vi "Vision Processing.vi"(4 "error in (no error)":errorcluster) -> ()   [LabVIEW 2019]
doc: "This VI runs in parallel to other tasks. It gets images from the camera, processes them for color or shape and use that information to affect robot behavior."
uses:
  <vilib>/Rock Robotics/WPI/Camera/WPI_CameraWhite Balance Values.ctl
  <vilib>/Rock Robotics/WPI/Camera/WPI_CameraFrameRate.ctl
  <vilib>/Rock Robotics/WPI/Camera/WPI_CameraImageSize.ctl
  Robot Global Data.vi
  <vilib>/Rock Robotics/Network Tables/NT Write Number.vi
  <vilib>/Rock Robotics/Network Tables/NT Read Number.vi
  <vilib>/Rock Robotics/Network Tables/NT Write Boolean.vi
panel:
  out "LimeLight":T1
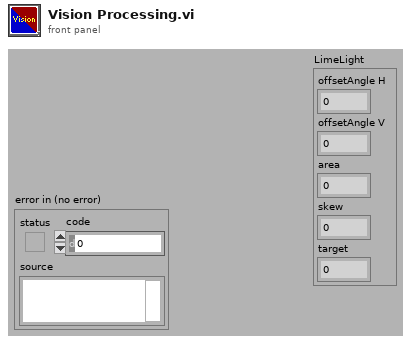
[diagram p1: front panel]
types:
  T1 = cluster{"offsetAngle H":dbl, "offsetAngle V":dbl, "area":dbl, "skew":dbl, "target":dbl}
  T2 = typedef "WPI_CameraImageSize.ctl" = enum16{"640x480", "320x240", "160x120", "Custom"}
  T3 = typedef "WPI_CameraFrameRate.ctl" = u32
  T4 = typedef "WPI_CameraWhite Balance Values.ctl" = enum16{"Auto", "Fixed indoor", "Fixed outdoor 1", "Fixed outdoor 2", "Fixed fluorescent 1", "Fixed fluorescent 2", "Hold current", "Custom"}
  T5 = typedef "WPI_DigitalInputDevRef.ctl" = cluster{"DevStatus":errorcluster, "DIO Channel":T6}
  T6 = typedef "FPGA_DIOChannel.ctl" = enum8{"DIO 0", "DIO 1", "DIO 2", "DIO 3", "DIO 4", "DIO 5", "DIO 6", "DIO 7", "DIO 8", "DIO 9", "DIO MXP 0", "DIO MXP 1", "DIO MXP 2", "DIO MXP 3", "DIO MXP 4", "DIO MXP 5", "DIO MXP 6", "DIO MXP 7", "DIO MXP 8", "DIO MXP 9", "DIO MXP 10", "DIO MXP 11", "DIO MXP 12", "DIO MXP 13", "DIO MXP 14", "DIO MXP 15", "SPI Port CS1", "SPI Port CS2", "SPI Port CS3", "SPI Port MISO", "SPI Port MOSI", "Invalid"}
  T7 = typedef "WPI_AnalogChannelDevRef.ctl" = cluster{"DevStatus":errorcluster, "Analog Channel":T8}
  T8 = typedef "FPGA_AIChannel.ctl" = enum8{"AI 0", "AI 1", "AI 2", "AI 3", "AI MXP 0", "AI MXP 1", "AI MXP 2", "AI MXP 3", "Invalid"}
  T9 = typedef "WPI_CameraDevRef.ctl" = cluster{"Camera Address":string, "CameraStatus":errorcluster}
  T10 = typedef "Image Type" = u32
  T11 = typedef "IMAQ Image.ctl" = refnum<image>
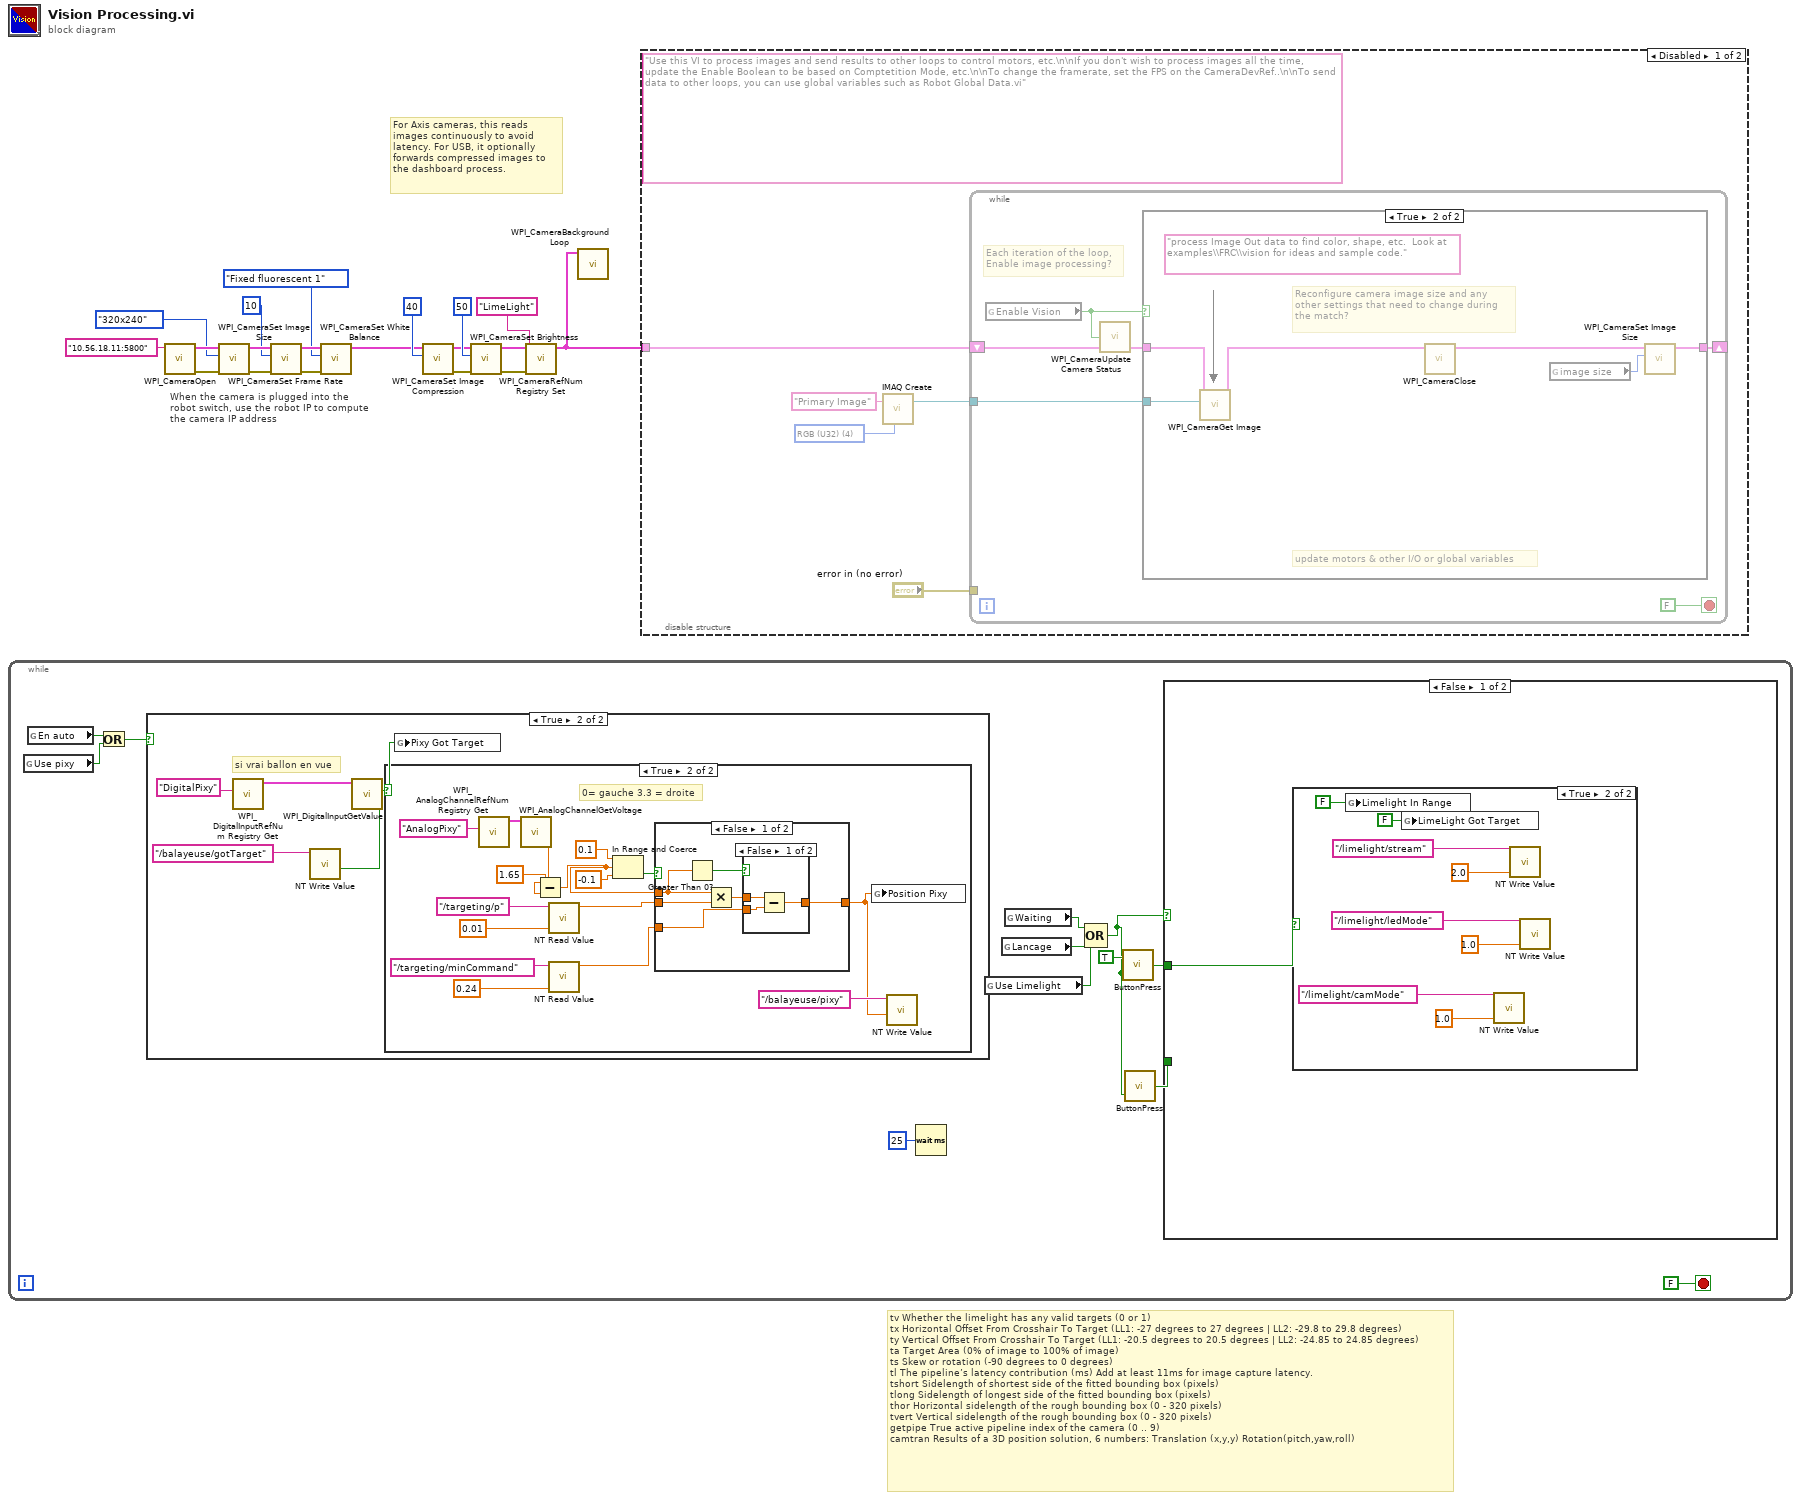
[diagram p0: block diagram]
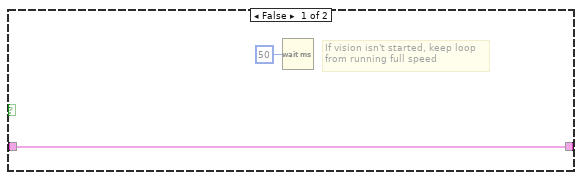
[diagram p2: hidden frame]
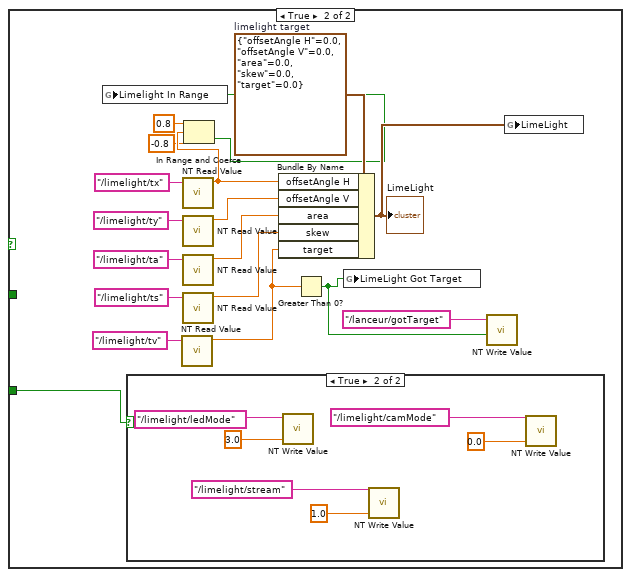
[diagram p5: hidden frame]
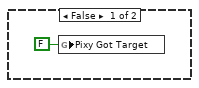
[diagram p7: hidden frame]
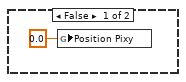
[diagram p8: hidden frame]
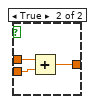
[diagram p9: hidden frame]
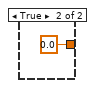
[diagram p10: hidden frame]
diagram:
  # "When the camera is plugged into the\nrobot switch, use the robot IP to compute\nthe camera IP address"
  # "For Axis cameras, this reads\nimages continuously to avoid\nlatency. For USB, it optionally\nforwards compressed images to\nthe dashboard process."
  # "tv\tWhether the limelight has any valid targets (0 or 1)\ntx\tHorizontal Offset From Crosshair To Target (LL1: -27 degrees to 27 degrees | LL2: -29.8 to 29.8 degrees)\nty\tVertical Offset From Crosshair To Target (LL1: -20.5 degrees to 20.5 degrees | LL2: -24.85 to 24.85 degrees)\nta\tTarget Area (0% of image to 100% of image)\nts\tSkew or rotation (-90 degrees to 0 degrees)\ntl\tThe pipeline’s latency contribution (ms) Add at least 11ms for image capture latency.\ntshort\tSidelength of shortest side of the fitted bounding box (pixels)\ntlong\tSidelength of longest side of the fitted bounding box (pixels)\nthor\tHorizontal sidelength of the rough bounding box (0 - 320 pixels)\ntvert\tVertical sidelength of the rough bounding box (0 - 320 pixels)\ngetpipe\tTrue active pipeline index of the camera (0 .. 9)\ncamtran\tResults of a 3D position solution, 6 numbers: Translation (x,y,y) Rotation(pitch,yaw,roll)"
  n1 = while {
    stop <- FALSE stop-if-true
    n2 = global read "Robot Global Data.vi" "Use pixy"() -> (w26:bool)
    n3 = global read "Robot Global Data.vi" "En auto"() -> (w25:bool)
    n4 = Or(x=w25, y=w26) -> (x .or. y?=w24:bool)
    n5 = case shown="True" w24 {
      frame False {
        n6 = global write "Robot Global Data.vi" "Pixy Got Target"(FALSE ("Pixy Got Target")) -> ()
      }
      frame True {
        # "si vrai ballon en vue"
        n7 = call <vilib>:"WPI_DigitalInputRefNum Registry Get.vi"("refnum name"="DigitalPixy") -> ("DigitalInputDevRef"=w69:T5)  [unwired: 9 in, 1 out]
        n8 = call <vilib>:"WPI_DigitalInputGetValue.vi"("DigitalInputDevRef"=w69) -> ("Value"=w67:bool)  [unwired: 8 in, 2 out]
        n9 = call-poly <vilib>:"NT Write Value.vi"("Boolean"=w67, "Name"="/balayeuse/gotTarget") -> ()  [unwired: 9 in, 1 out]
        n10 = case shown="True" w67 {
          frame False {
            n11 = global write "Robot Global Data.vi" "Position Pixy"(0.0 ("Position Pixy")) -> ()
          }
          frame True {
            # "0= gauche 3.3 = droite"
            n12 = call <vilib>:"WPI_AnalogChannelRefNum Registry Get.vi"("refnum name"="AnalogPixy") -> ("AIDeviceRef"=w86:T7)  [unwired: 9 in, 1 out]
            n13 = call <vilib>:"WPI_AnalogChannelGetVoltage.vi"("AIDeviceRef"=w86) -> ("Voltage"=w81:dbl)  [unwired: 8 in, 2 out]
            n14 = Subtract(x=w81, y=1.65) -> (x-y=w79:dbl)
            n15 = call-poly <vilib>:"NT Read Value.vi"("Default Value"=0.01, "Name"="/targeting/p") -> ("Numeric"=w72:dbl)  [unwired: 8 in, 1 out]
            n16 = call-poly <vilib>:"NT Read Value.vi"("Default Value"=0.24, "Name"="/targeting/minCommand") -> ("Numeric"=w71:dbl)  [unwired: 8 in, 1 out]
            n17 = In Range and Coerce(upper limit=0.1, x=w79, lower limit=-0.1) -> (In Range?=w82:bool)  [unwired: 1 out]
            n18 = case shown="False" w82 {
              tunnel: [w90 0.0] -> w77
              tunnel: w79 -> [w89 _]
              tunnel: w72 -> [w88 _]
              tunnel: w71 -> [w87 _]
              frame False {
                n19 = Greater Than 0?(x=w89) -> (x > 0?=w92:bool)
                n20 = Multiply(x=w89, y=w88) -> (x*y=w91:dbl)
                n21 = case shown="False" w92 {
                  tunnel: w91 -> [w95 w98]
                  tunnel: w87 -> [w94 w97]
                  tunnel: [w93 w96] -> w90
                  frame False {
                    n22 = Subtract(x=w95, y=w94) -> (x-y=w93:dbl)
                  }
                  frame True {
                    n23 = Add(x=w98, y=w97) -> (x+y=w96:dbl)
                  }
                }
              }
              frame True {
              }
            }
            n24 = global write "Robot Global Data.vi" "Position Pixy"(w77) -> ()
            n25 = call-poly <vilib>:"NT Write Value.vi"("Numeric"=w77, "Name"="/balayeuse/pixy") -> ()  [unwired: 9 in, 1 out]
          }
        }
        n26 = global write "Robot Global Data.vi" "Pixy Got Target"(w67) -> ()
      }
    }
    n27 = Wait (ms)(milliseconds to wait=u32 25) -> ()  [unwired: 1 out]
    n28 = global read "Robot Global Data.vi" "Use Limelight"() -> (w20:bool)
    n29 = global read "Robot Global Data.vi" "Lancage"() -> (w23:bool)
    n30 = global read "Robot Global Data.vi" "Waiting"() -> (w22:bool)
    n31 = Compound Arithmetic op=OR(w22, w23, w20) -> (w21:bool)
    n32 = call "ButtonPress.vi"("Input"=w21, "Falling Edge?"=TRUE) -> ("Output"=w28:bool)
    n33 = call "ButtonPress.vi"("Input"=w21) -> ("Output"=w27:bool)  [unwired: 1 in]
    n34 = case shown="False" w21 {
      tunnel: w28 -> [w32 _]
      tunnel: w27 -> [_ w47]
      frame False {
        n35 = case shown="True" w32 {
          frame False {
          }
          frame True {
            n36 = global write "Robot Global Data.vi" "Limelight In Range"(FALSE ("LimeLight Got Target")) -> ()
            n37 = global write "Robot Global Data.vi" "LimeLight Got Target"(FALSE ("LimeLight Got Target")) -> ()
            n38 = call-poly <vilib>:"NT Write Value.vi"("Numeric"=1.0, "Name"="/limelight/camMode") -> ()  [unwired: 9 in, 1 out]
            n39 = call-poly <vilib>:"NT Write Value.vi"("Numeric"=2.0, "Name"="/limelight/stream") -> ()  [unwired: 9 in, 1 out]
            n40 = call-poly <vilib>:"NT Write Value.vi"("Numeric"=1.0, "Name"="/limelight/ledMode") -> ()  [unwired: 9 in, 1 out]
          }
        }
      }
      frame True {
        w54 = T1 {"offsetAngle H"=0.0, "offsetAngle V"=0.0, "area"=0.0, "skew"=0.0, "target"=0.0}  # limelight target
        n41 = case shown="True" w47 {
          frame False {
          }
          frame True {
            n42 = call-poly <vilib>:"NT Write Value.vi"("Numeric"=3.0, "Name"="/limelight/ledMode") -> ()  [unwired: 9 in, 1 out]
            n43 = call-poly <vilib>:"NT Write Value.vi"("Numeric"=1.0, "Name"="/limelight/stream") -> ()  [unwired: 9 in, 1 out]
            n44 = call-poly <vilib>:"NT Write Value.vi"("Numeric"=0.0, "Name"="/limelight/camMode") -> ()  [unwired: 9 in, 1 out]
          }
        }
        n45 = call-poly <vilib>:"NT Read Value.vi"("Name"="/limelight/tv") -> ("Numeric"=w48:dbl)  [unwired: 9 in, 1 out]
        n46 = call-poly <vilib>:"NT Read Value.vi"("Name"="/limelight/tx") -> ("Numeric"=w44:dbl)  [unwired: 9 in, 1 out]
        n47 = call-poly <vilib>:"NT Read Value.vi"("Name"="/limelight/ty") -> ("Numeric"=w53:dbl)  [unwired: 9 in, 1 out]
        n48 = call-poly <vilib>:"NT Read Value.vi"("Name"="/limelight/ta") -> ("Numeric"=w52:dbl)  [unwired: 9 in, 1 out]
        n49 = call-poly <vilib>:"NT Read Value.vi"("Name"="/limelight/ts") -> ("Numeric"=w51:dbl)  [unwired: 9 in, 1 out]
        n50 = In Range and Coerce(upper limit=0.8, x=w44, lower limit=-0.8) -> (In Range?=w41:bool)  [unwired: 1 out]
        n51 = global write "Robot Global Data.vi" "Limelight In Range"(w41) -> ()
        n52 = Bundle By Name(cluster=w54, "offsetAngle H"=w44, "offsetAngle V"=w53, "area"=w52, "skew"=w51, "target"=w48) -> (w49:T1)
        "LimeLight" <- w49
        n53 = Greater Than 0?(x=w48) -> (x > 0?=w45:bool)
        n54 = global write "Robot Global Data.vi" "LimeLight Got Target"(w45) -> ()
        n55 = call-poly <vilib>:"NT Write Value.vi"("Boolean"=w45, "Name"="/lanceur/gotTarget") -> ()  [unwired: 9 in, 1 out]
        n56 = global write "Robot Global Data.vi" "LimeLight"(w49) -> ()
      }
    }
  }
  n57 = call <vilib>:"WPI_CameraOpen.vi"("Camera Address"="10.56.18.11:5800" ("format string")) -> ("error out"=w11:errorcluster, "CameraDevRef"=w12:T9)  [unwired: 1 in, 8 out]
  n58 = call <vilib>:"WPI_CameraSet Image Size.vi"("error in (no error)"=w11, "Image Size"=WPI_CameraImageSize."320x240", "CameraDevRef"=w12) -> ("error out"=w10:errorcluster, "CameraDevRef Out"=w13:T9)  [unwired: 1 in, 6 out]
  n59 = call <vilib>:"WPI_CameraSet Frame Rate.vi"("error in (no error)"=w10, "Frame Rate (fps)"=T3 10, "CameraDevRef"=w13) -> ("error out"=w9:errorcluster, "CameraDevRef Out"=w14:T9)  [unwired: 7 out]
  n60 = call <vilib>:"WPI_CameraSet White Balance.vi"("error in (no error)"=w9, "White Balance"=WPI_CameraWhite_Balance_Values."Fixed fluorescent 1", "CameraDevRef"=w14) -> ("CameraDevRef Out"=w1:T9)  [unwired: 1 in, 7 out]
  n61 = call <vilib>:"WPI_CameraSet Image Compression.vi"("Compression"=40, "CameraDevRef"=w1) -> ("error out"=w8:errorcluster, "CameraDevRef Out"=w15:T9)  [unwired: 1 in, 7 out]
  n62 = call <vilib>:"WPI_CameraSet Brightness.vi"("error in (no error)"=w8, "Brightness"=50, "CameraDevRef"=w15) -> ("error out"=w6:errorcluster, "CameraDevRef Out"=w7:T9)  [unwired: 1 in, 6 out]
  n63 = call <vilib>:"WPI_CameraRefNum Registry Set.vi"("error in (no error)"=w6, "refnum name"="LimeLight", "CameraDevRef"=w7) -> ("CameraDevRef"=w19:T9)  [unwired: 1 in, 7 out]
  n64 = call <vilib>:"WPI_CameraBackground Loop.vi"("CameraDevRef"=w19) -> ()  [unwired: 11 in]
  n65 = disable-structure shown="Disabled" {
    disable-tunnel: w19 -> [w102 _]
    frame Disabled {
      (unwired) "Use this VI to process images and send results to other loops to control motors, etc.\n\nIf you don't wish to process images all the time, update the Enable Boolean to be based on Comptetition Mode, etc.\n\nTo change the framerate, set the FPS on the CameraDevRef..\n\nTo send data to other loops, you can use global variables such as Robot Global Data.vi"
      w105 = T10 4 items=["Grayscale (U8)", "Grayscale (I16)", "Grayscale (SGL)", "Complex (CSG)", "RGB (U32)", "HSL (U32)", "RGB (U64)"] ("Image Type")
      n66 = call "IMAQ Create"("Image Name"="Primary Image", "Image Type"=w105) -> ("New Image"=w103:T11)  [unwired: 2 in, 2 out]
      n67 = while {
        shift-right: [w110] -> w101
        shift-left: w102 -> [w108]
        tunnel: w103 -> [w109]
        tunnel: "error in (no error)" -> [_]
        stop <- FALSE stop-if-true
        # "Each iteration of the loop,\nEnable image processing?"
        n68 = global read "Robot Global Data.vi" "Enable Vision"() -> (w106:bool)
        n69 = call <vilib>:"WPI_CameraUpdate Camera Status.vi"("CameraDevRef In"=w108, "Enable Vision"=w106) -> ("CameraDevRef Out"=w107:T9)  [unwired: 3 in]
        n70 = case shown="True" w106 {
          tunnel: w109 -> [_ w117]
          tunnel: [w113 w118] -> w110
          tunnel: w107 -> [w113 w115]
          frame False {
            # "If vision isn't started, keep loop\nfrom running full speed"
            n71 = Wait (ms)(milliseconds to wait=u32 50) -> ()  [unwired: 1 out]
          }
          frame True {
            (unwired) "process Image Out data to find color, shape, etc.  Look at examples\\FRC\\vision for ideas and sample code."
            # "update motors & other I/O or global variables"
            # "Reconfigure camera image size and any\nother settings that need to change during\nthe match?"
            n72 = call <vilib>:"WPI_CameraGet Image.vi"("Image"=w117, "CameraDevRef"=w115) -> ("CameraDevRef Out"=w114:T9)  [unwired: 1 in, 8 out]
            n73 = global read "Robot Global Data.vi" "image size"() -> (w116:T2)
            n74 = call <vilib>:"WPI_CameraSet Image Size.vi"("Image Size"=w116, "CameraDevRef"=w114) -> ("CameraDevRef Out"=w118:T9)  [unwired: 2 in, 7 out]
          }
        }
      }
      n75 = call <vilib>:"WPI_CameraClose.vi"("CameraDevRef"=w101) -> ()  [unwired: 1 in, 10 out]
    }
    frame Enabled {
    }
  }
